vi "validate line configuration.vi"(7 "EthernetIP configuration":refnum<class "EthernetIP configuration.lvclass">, 11 "line in":T1) -> (1 "valid?":bool, 2 "problem":string, 3 "line out":T1)   [LabVIEW 2013, in "EthernetIP editor node.lvclass"]
uses:
  EthernetIP editor node.lvclass
  table line.ctl
  <vilib>/NI/TBM Modules/Ethernet IP/channel/EthernetIP Channel.lvclass
  <vilib>/NI/TBM Modules/Ethernet IP/configuration/EthernetIP configuration.lvclass
  <vilib>/NI/TBM Modules/Ethernet IP/channel/EthernetIP Channel.lvclass/EthernetIP Channel.ctl
  <vilib>/NI/Tag Bus/tag/tag descriptor.lvclass/tag descriptor.ctl
  <vilib>/NI/Tag Bus Module Framework/channel/TBM channel.lvclass/TBM channel.ctl
  <vilib>/NI/TBM Modules/Ethernet IP/configuration/EthernetIP configuration.lvclass/EthernetIP configuration.ctl
  <vilib>/NI/TBM Modules/Ethernet IP/channel/Read byte index.vi
  <vilib>/NI/TBM Modules/Ethernet IP/channel/Read Instance ID.vi
  <vilib>/NI/TBM Modules/Ethernet IP/configuration/read eip channels.vi
  <vilib>/NI/TBM Modules/Ethernet IP/configuration/Read assemblies.vi
  <vilib>/NI/Tag Bus/tag/read tag name.vi
  <vilib>/NI/Tag Bus Module Framework/channel/Read channel classification.vi
  <vilib>/NI/Tag Bus/tag/tag descriptor.lvclass
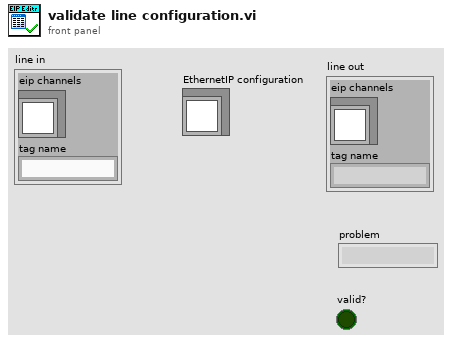
[diagram p1: front panel]
types:
  T1 = typedef "EthernetIP editor node.lvclass/table line.ctl" = cluster{"eip channels":refnum<class "EthernetIP Channel.lvclass">, "tag name":string}
  T2 = typedef "TBM channel.lvclass/channel classification.ctl" = enum16{"input data", "output data", "processing parameter", "processing result"}
  T3 = typedef "EthernetIP configuration.lvclass/assembly definition.ctl" = cluster{"name":string, "Instance ID":u32, "Type":T4, "Size (elements)":u32, "big endian?":bool, "data type":T5}
  T4 = typedef "EthernetIP configuration.lvclass/assembly type.ctl" = enum32{"Producing", "Consuming"}
  T5 = typedef "tag bus.lvlib/tag descriptor.lvclass/Data Type.ctl" = enum16{"Double", "Single", "I64", "I32", "I16", "I8", "U64", "U32", "U16", "U8", "Boolean", "String", "Array of Double", "Array of Single", "Array of I64", "Array of I32", "Array of I16", "Array of I8", "Array of U64", "Array of U32", "Array of U16", "Array of U8", "Array of Boolean", "Array of String"}
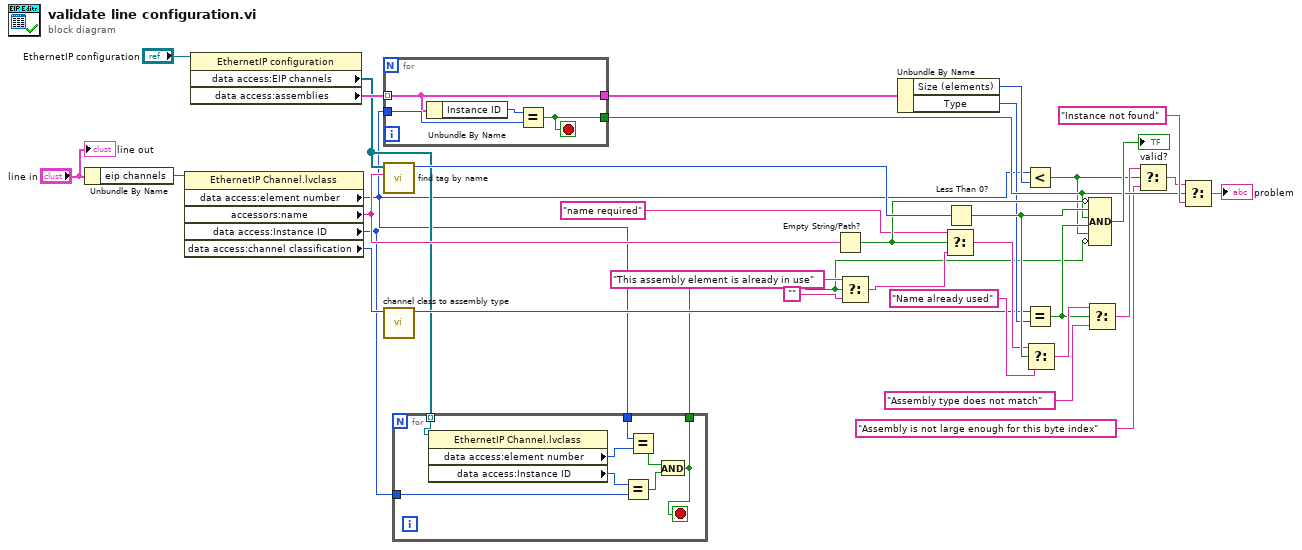
[diagram p0: block diagram]
diagram:
  n1 = Unbundle By Name("line in") -> ("eip channels"=w33:refnum<class "EthernetIP Channel.lvclass">)
  n2 = property class="EthernetIP Channel.lvclass"(reference=w33) -> ("data access:element number"=w6:i32, "accessors:name"=w31:string, "data access:Instance ID"=w5:u32, "data access:channel classification"=w20:T2)  [unwired: 1 in, 2 out]
  n3 = property class="EthernetIP configuration"(reference="EthernetIP configuration") -> ("data access:EIP channels"=w7:refnum<class "EthernetIP Channel.lvclass">[], "data access:assemblies"=w28:T3[])  [unwired: 1 in, 2 out]
  n4 = for {
    tunnel: w28 -> [w36] mode=indexing
    tunnel: w5 -> [w37]
    tunnel: [w36] -> w16
    tunnel: [w35] -> w21
    stop <- w35 stop-if-true
    n5 = Unbundle By Name(w36) -> ("Instance ID"=w38:u32)
    n6 = Equal?(x=w38, y=w37) -> (x = y?=w35:bool)
  }
  n7 = call <vilib>:"find tag by name.vi"("name"=w31, "tags in"=w7) -> ("index"=w29:i32)  [unwired: 9 in]
  n8 = call <vilib>:"channel class to assembly type.vi"("channel classification"=w20) -> ("assembly types"=w11:T4)  [unwired: 10 in]
  n9 = for {
    tunnel: w7 -> [w46] mode=indexing
    tunnel: w6 -> [w44]
    tunnel: w5 -> [w42]
    tunnel: [w39] -> w1
    stop <- w39 stop-if-true
    n10 = property class="EthernetIP Channel.lvclass"(reference=w46) -> ("data access:element number"=w45:i32, "data access:Instance ID"=w43:u32)  [unwired: 1 in, 2 out]
    n11 = Equal?(x=w43, y=w42) -> (x = y?=w40:bool)
    n12 = Equal?(x=w44, y=w45) -> (x = y?=w41:bool)
    n13 = And(x=w41, y=w40) -> (x .and. y?=w39:bool)
  }
  n14 = Empty String/Path?(string/path=w31) -> (empty?=w27:bool)
  n15 = Select(t="This assembly element is already in use", s=w1, f="") -> (s? t:f=w3:string)
  n16 = Unbundle By Name(w16) -> ("Size (elements)"=w9:u32, "Type"=w12:T4)
  n17 = Select(t="name required", s=w27, f=w3) -> (s? t:f=w25:string)
  n18 = Less Than 0?(x=w29) -> (x < 0?=w26:bool)
  n19 = Less?(x=w6, y=w9) -> (x < y?=w8:bool)
  n20 = Equal?(x=w11, y=w12) -> (x = y?=w10:bool)
  n21 = Select(t=w25, s=w26, f="Name already used") -> (s? t:f=w15:string)
  n22 = Select(t=w15, s=w10, f="Assembly type does not match") -> (s? t:f=w17:string)
  n23 = Compound Arithmetic op=AND(invert w27, w26, w21, w10, w8, invert w1) -> (→"valid?":bool)
  n24 = Select(t=w17, s=w8, f="Assembly is not large enough for this byte index") -> (s? t:f=w14:string)
  n25 = Select(t=w14, s=w21, f="Instance not found") -> (s? t:f=→"problem":string)
  "line out" <- "line in"
